vi "rcv_rsvp.vi"(2 "error in (no error)":errorcluster) -> (0 "error out":errorcluster, 1 "response string":string)   [LabVIEW 2017]
doc: "Reveive Response\nGet the return string from the Cornerstone"
uses:
  m_globals.vi
panel:
  out "null string":bool
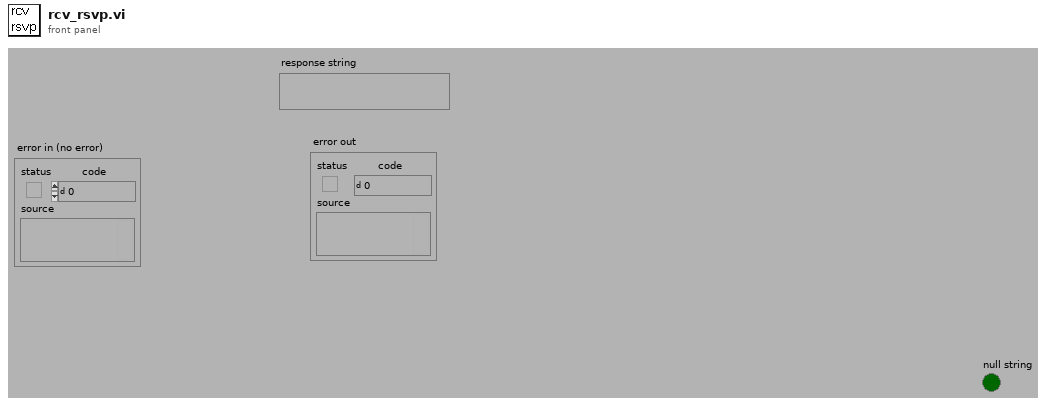
[diagram p1: front panel]
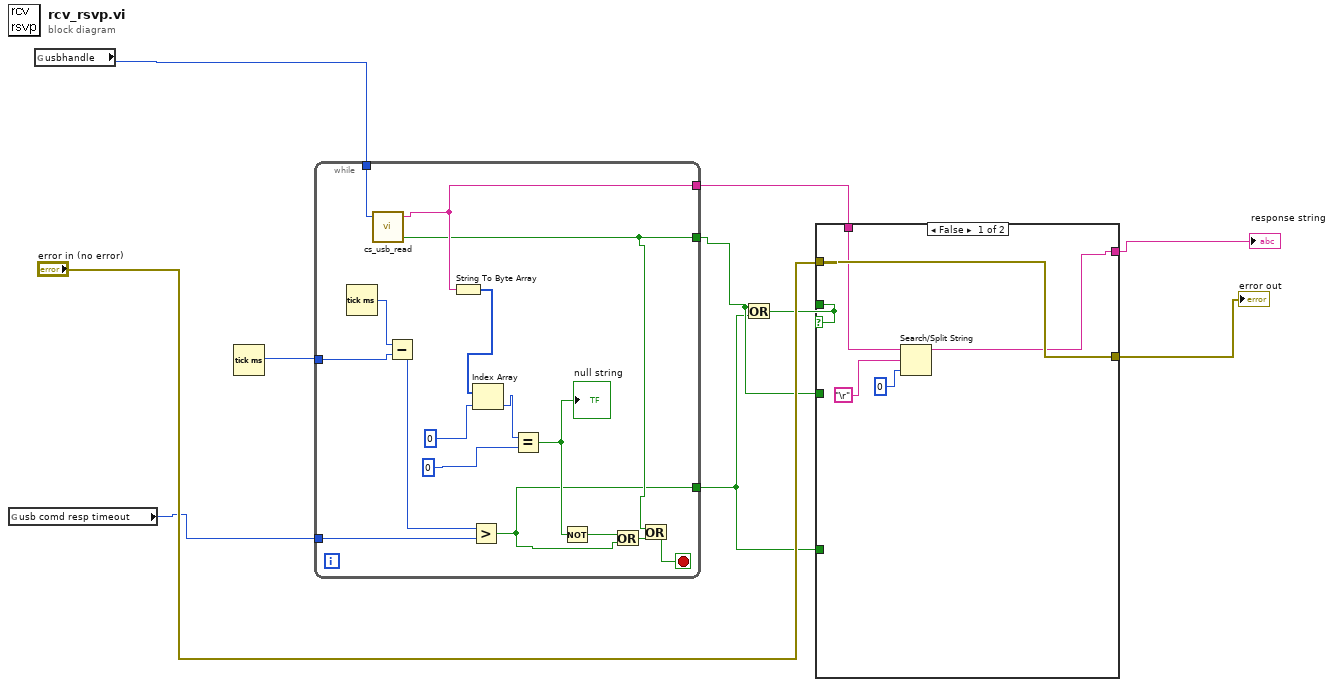
[diagram p0: block diagram]
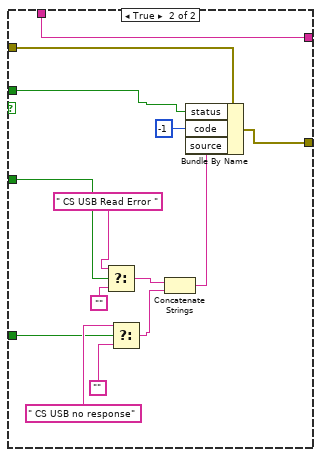
[diagram p2: hidden frame]
diagram:
  n1 = global read "m_globals.vi" "usb comd resp timeout"() -> (w4:i32)
  n2 = global read "m_globals.vi" "usbhandle"() -> (w10:i32)
  n3 = Tick Count (ms)() -> (millisecond timer value=w5:u32)
  n4 = while {
    tunnel: w10 -> [w26]
    tunnel: [w16] -> w6
    tunnel: w5 -> [w12]
    tunnel: [w20] -> w2
    tunnel: w4 -> [w15]
    tunnel: [w13] -> w3
    stop <- w17 stop-if-true
    n5 = Tick Count (ms)() -> (millisecond timer value=w11:u32)
    n6 = call "cs_usb_read.vi"("handle"=w26) -> ("Error"=w16:bool, "string"=w20:string)  [unwired: 3 in]
    n7 = Subtract(x=w11, y=w12) -> (x-y=w21:u32)
    n8 = String To Byte Array(string=w20) -> (unsigned byte array=w25:u8[])
    n9 = Greater?(x=w21, y=w15) -> (0:w13:bool)
    n10 = Index Array(array=w25, index=0 ("offset (0)")) -> (element=w22:u8)
    n11 = Equal?(x=w22, y=u8 0 ("length (rest)")) -> (x = y?=w14:bool)
    "null string" <- w14
    n12 = Not(x=w14) -> (.not. x?=w19:bool)
    n13 = Or(x=w19, y=w13) -> (x .or. y?=w18:bool)
    n14 = Or(x=w16, y=w18) -> (x .or. y?=w17:bool)
  }
  n15 = Or(x=w6, y=w3) -> (x .or. y?=w7:bool)
  n16 = case shown="False" w7 {
    tunnel: "error in (no error)" -> [w31 w44]
    tunnel: [w31 w45] -> w9
    tunnel: w7 -> [_ w42]
    tunnel: w6 -> [_ w41]
    tunnel: w3 -> [_ w33]
    tunnel: w2 -> [w30 w32]
    tunnel: [w28 w32] -> w1
    frame False {
      n17 = Search/Split String(string=w30, search string/char (-)="\r", offset (0)=0) -> (substring before match=w28:string)  [unwired: 2 out]
    }
    frame True {
      n18 = Select(t=" CS USB Read Error " ("source"), s=w41, f="") -> (s? t:f=w36:string)
      n19 = Select(t=" CS USB no response" ("source"), s=w33, f="") -> (s? t:f=w35:string)
      n20 = Concatenate Strings(w36, w35) -> (w37:string)
      n21 = Bundle By Name(cluster=w44, "status"=w42, "code"=-1, "source"=w37) -> (w45:errorcluster)
    }
  }
  "error out" <- w9
  "response string" <- w1
